vi "Configure Arbitrary Waveform Sequence.vi"(6 "Sequence Iterations (1)":dbl[](array[numeric]) min=1.0 max=32768.0, 7 "Enable Sequence Segment (T: Enable)":bool[](array[boolean])=[TRUE], 8 "error in (no error)":errorcluster, 9 "Start Sequence Step (0: Count)":u16[](array[ring]) items=["Count", "Trigger Edge", "Trigger Level"], 10 "Arbitrary Sequence Waveform Name":string[](array[string]), 11 "VISA resource name":refnum<visa-resource-name>) -> (0 "error out":errorcluster, 3 "VISA resource name out":refnum<visa-resource-name>)   [LabVIEW 2015, in "Fluke 28x Series.lvlib"]
doc: "Configures a sequence of waveforms consisting only of arbitrary waveforms."
uses:
  <instrlib>/Fluke 28x Series/Fluke 28x Series.lvlib
panel:
  # "Start Sequence Step on Count"
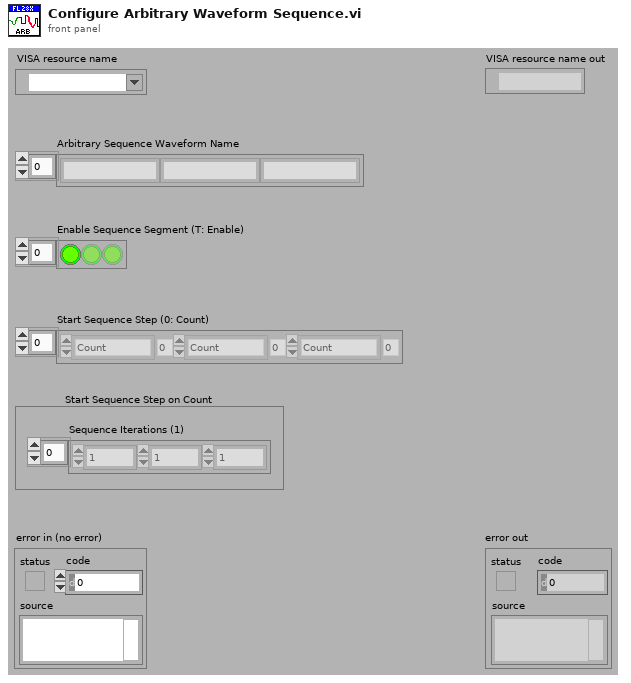
[diagram p1: front panel]
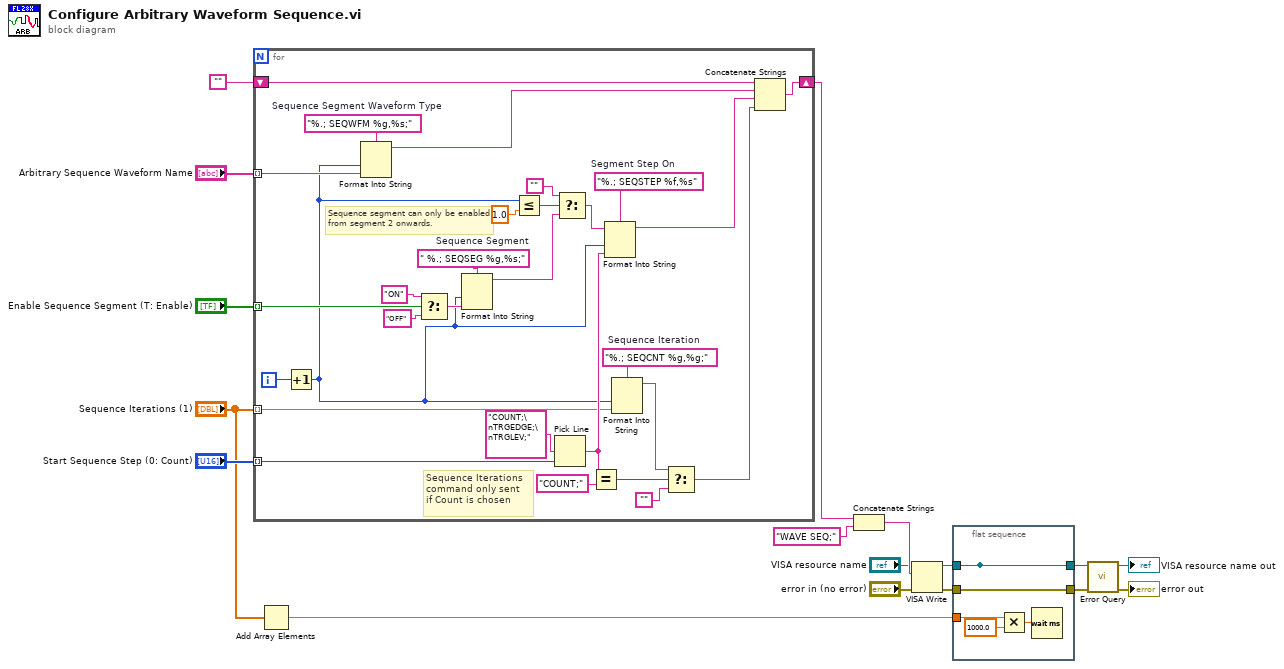
[diagram p0: block diagram]
diagram:
  n1 = for {
    tunnel: "Arbitrary Sequence Waveform Name" -> [w44] mode=indexing
    tunnel: "Enable Sequence Segment (T: Enable)" -> [w33] mode=indexing
    tunnel: "Start Sequence Step (0: Count)" -> [w24] mode=indexing
    shift-right: [w19] -> w11
    shift-left: "" -> [w20]
    tunnel: "Sequence Iterations (1)" -> [w18] mode=indexing
    i -> [w46]
    w29 = "%.; SEQCNT %g,%g;"  # Sequence Iteration
    w38 = "%.; SEQSTEP %f,%s"  # Segment Step On
    w37 = " %.; SEQSEG %g,%s;"  # Sequence Segment
    w45 = "%.; SEQWFM %g,%s;"  # Sequence Segment Waveform Type
    # "Sequence Iterations\ncommand only sent\nif Count is chosen"
    # "Sequence segment can only be enabled from segment 2 onwards."
    n2 = Increment(x=w46) -> (x+1=w21:i32)
    n3 = Format Into String(format string=w45, w21, w44) -> (resulting string=w32:string)  [unwired: 2 in, 1 out]
    n4 = Select(t="ON", s=w33, f="OFF") -> (s? t:f=w36:string)
    n5 = Format Into String(format string=w37, w21, w36) -> (resulting string=w41:string)  [unwired: 2 in, 1 out]
    n6 = Less Or Equal?(x=w21, y=1.0) -> (x <= y?=w40:bool)
    n7 = Pick Line(multi-line string="COUNT;\nTRGEDGE;\nTRGLEV;", line index=w24) -> (output string=w23:string)  [unwired: 1 in]
    n8 = Select(t="", s=w40, f=w41) -> (s? t:f=w43:string)
    n9 = Equal?(x=w23, y="COUNT;") -> (x = y?=w27:bool)
    n10 = Format Into String(format string=w38, initial string=w43, w21, w23) -> (resulting string=w31:string)  [unwired: 1 in, 1 out]
    n11 = Format Into String(format string=w29, w21, w18) -> (resulting string=w30:string)  [unwired: 2 in, 1 out]
    n12 = Select(t=w30, s=w27, f="") -> (s? t:f=w22:string)
    n13 = Concatenate Strings(w20, w32, w31, w22) -> (w19:string)
  }
  n14 = Add Array Elements(numeric array="Sequence Iterations (1)") -> (sum=w1:dbl)
  n15 = Concatenate Strings(w11, "WAVE SEQ;" ("string")) -> (w9:string)
  n16 = VISA Write(VISA resource name="VISA resource name", write buffer=w9, error in (no error)="error in (no error)") -> (VISA resource name out=w5:refnum<visa-resource-name>, error out=w3:errorcluster)  [unwired: 1 out]
  n17 = flat-sequence {
    tunnel: [w51] -> _
    tunnel: w5 -> [w51]
    tunnel: [w51] -> w4
    tunnel: w3 -> [w50]
    tunnel: [w50] -> w2
    tunnel: w1 -> [w49]
    frame #0 {
      n18 = Multiply(x=w49, y=1000.0) -> (x*y=w47:dbl)
      n19 = Wait (ms)(milliseconds to wait=w47) -> ()  [unwired: 1 out]
    }
  }
  n20 = call <instrlib>:"Error Query.vi"("error in (no error)"=w2, "VISA resource name"=w4) -> ("error out"=→"error out":errorcluster, "VISA resource name out"=→"VISA resource name out":refnum<visa-resource-name>)  [unwired: 6 in, 2 out]
